vi "and.vi"() -> ()   [LabVIEW 2020]
panel:
  out "x .and. y? 2":i32 format="%b"
  in  "Numeric 2":u8 format="%b"
  in  "Numeric":u8 format="%b"
  out "x .and. y?":bool
  in  "Boolean 2":bool
  in  "Boolean":bool
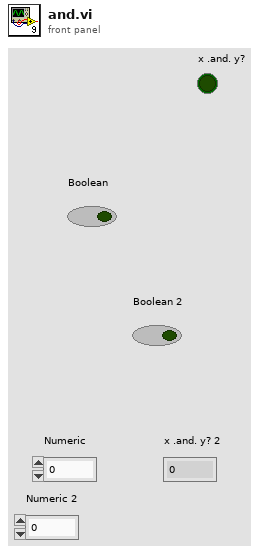
[diagram p1: front panel]
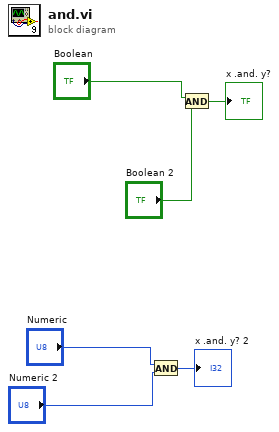
[diagram p0: block diagram]
diagram:
  n1 = And(x="Numeric", y="Numeric 2") -> (x .and. y?=→"x .and. y? 2":u8)
  n2 = And(x="Boolean", y="Boolean 2") -> (x .and. y?=→"x .and. y?":bool)
